vi "loop20 (Kopie).vi"() -> ()   [LabVIEW 2010]
uses:
  <vilib>/Utility/file.llb/Write To Spreadsheet File (DBL).vi
  <vilib>/Analysis/NI_AALBase.lvlib
panel:
  out "Phasen Error":dbl
  out "Phasen Mean":dbl
  out "Amplituden Error":dbl
  out "Amplituden Mean":dbl
  out "Phasen":dbl[](array[numeric])
  out "Amplituden":dbl[](array[numeric])
  out "data X":dbl format="%#_6e"
  out "data Y":dbl
  in  "mode (0)":i16
  in  "address string":string="19"
  out "Counter":dbl[](array[numeric])
  in  "Path":path
  out "error out":errorcluster
  in  "error in (no error)":errorcluster
  in  "Start":dbl format="%.2f"
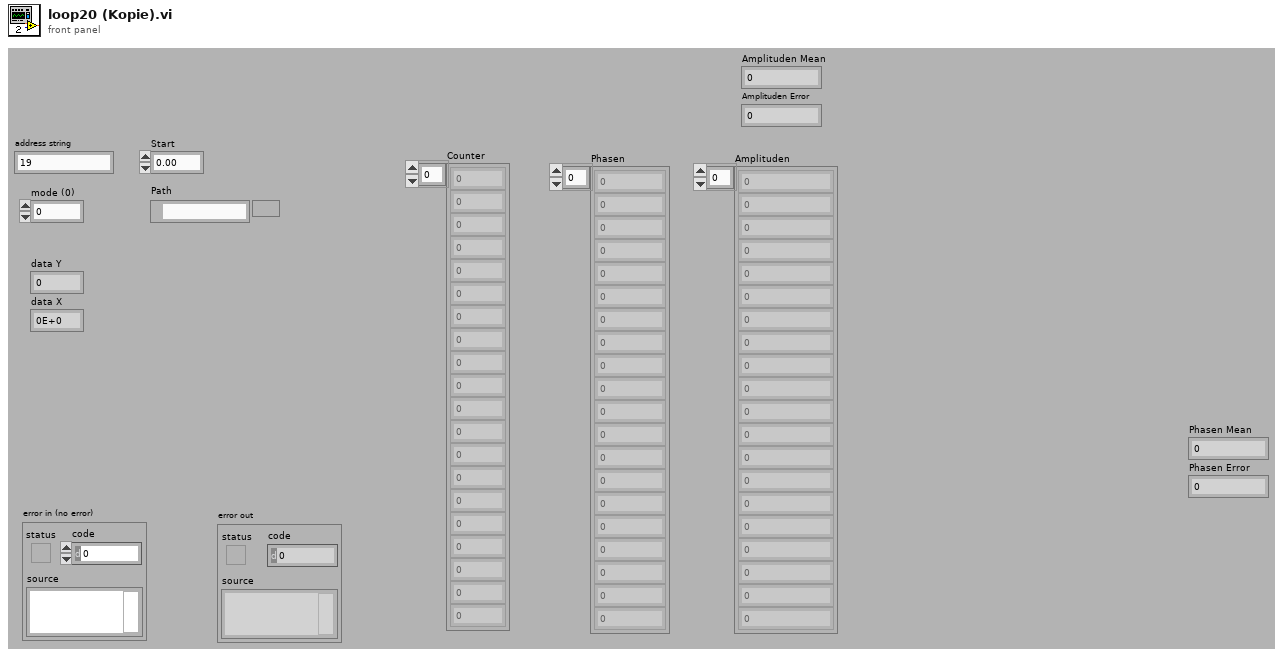
[diagram p1: front panel]
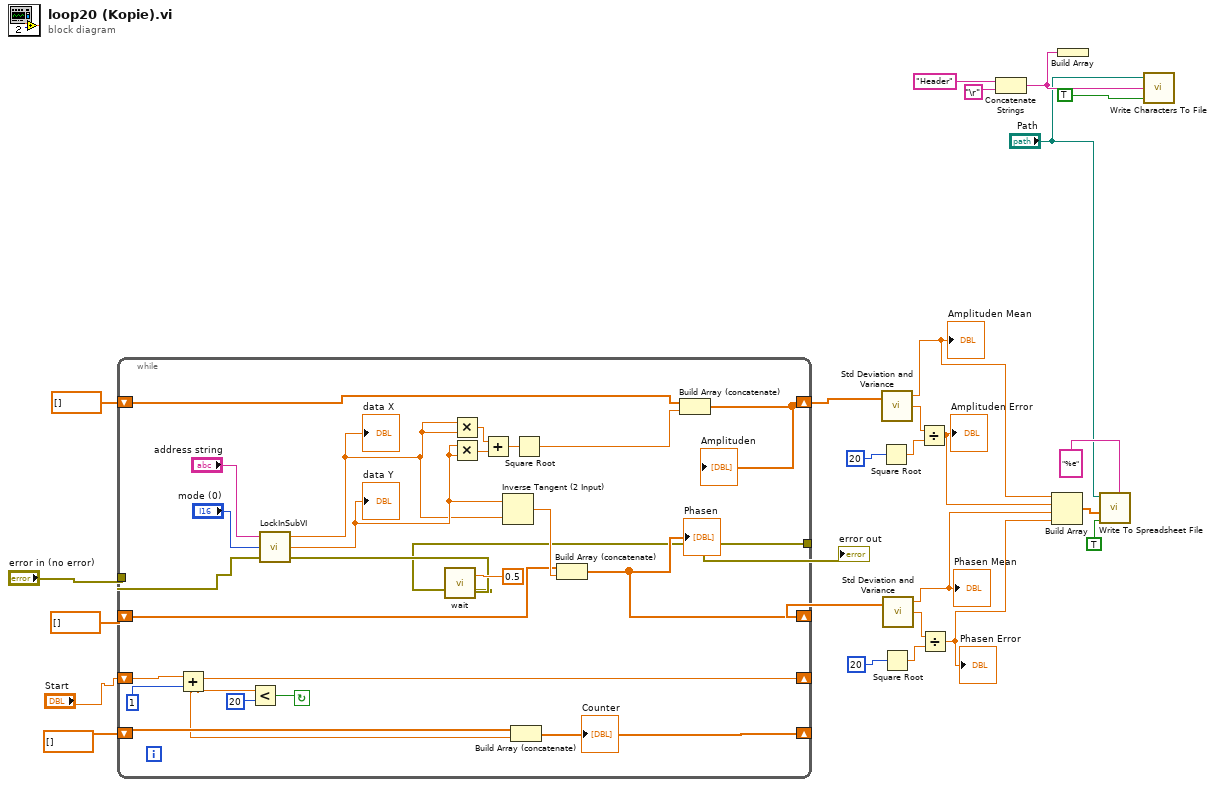
[diagram p0: block diagram]
diagram:
  n1 = while {
    tunnel: "error in (no error)" -> [w32]
    tunnel: [w33] -> w25
    shift-right: [w27] -> _
    shift-left: "Start" -> [w49]
    shift-right: [w28] -> _
    shift-left: dbl[] [] -> [w29]
    shift-right: [w39] -> w16
    shift-left: dbl[] [] -> [w40]
    shift-right: [w36] -> w9
    shift-left: dbl[] [] -> [w37]
    stop <- w30 continue-if-true
    n2 = Add(x=w49, y=1) -> (x+y=w27:dbl)
    n3 = Less?(x=w27, y=20) -> (x < y?=w30:bool)
    n4 = call "LockInSubVI.vi"("error in"=w32, "mode (0)"="mode (0)", "address string"="address string") -> ("error out 2"=w34:errorcluster, "data Y"=w43:dbl, "data X"=w42:dbl)
    "data Y" <- w43
    "data X" <- w42
    n5 = call "wait.vi"("error in"=w34, "Wartezeit in Sek"=0.5) -> ("error out"=w33:errorcluster)  [unwired: 1 in]
    n6 = Multiply(x=w42, y=w42) -> (x*y=w46:dbl)
    n7 = Multiply(x=w43, y=w43) -> (x*y=w45:dbl)
    n8 = Add(x=w46, y=w45) -> (x+y=w44:dbl)
    n9 = Inverse Tangent (2 Input)(1:w42, 2:w43) -> (0:w38:dbl)
    n10 = Build Array (concatenate)(w29, w27) -> (w28:dbl[])
    "Counter" <- w28
    n11 = Square Root(x=w44) -> (sqrt(x)=w41:dbl)
    n12 = Build Array (concatenate)(w37, w38) -> (w36:dbl[])
    "Phasen" <- w36
    n13 = Build Array (concatenate)(w40, w41) -> (w39:dbl[])
    "Amplituden" <- w39
  }
  "error out" <- w25
  n14 = Square Root(x=20) -> (sqrt(x)=w13:dbl)
  n15 = call <vilib>:"Std Deviation and Variance.vi"("X"=w16) -> ("mean"=w6:dbl, "standard deviation"=w15:dbl)  [unwired: 1 in, 1 out]
  "Amplituden Mean" <- w6
  n16 = Square Root(x=20) -> (sqrt(x)=w10:dbl)
  n17 = call <vilib>:"Std Deviation and Variance.vi"("X"=w9) -> ("mean"=w4:dbl, "standard deviation"=w12:dbl)  [unwired: 1 in, 1 out]
  "Phasen Mean" <- w4
  n18 = Divide(x=w15, y=w13) -> (x/y=w5:dbl)
  "Amplituden Error" <- w5
  n19 = Divide(x=w12, y=w10) -> (x/y=w3:dbl)
  "Phasen Error" <- w3
  n20 = Concatenate Strings("Header", "\r") -> (w21:string)
  n21 = Build Array(w6, w5, w4, w3) -> (w2:dbl[])
  n22 = Build Array(w21) -> ()  [unwired: 1 out]
  n23 = call-poly <vilib>:"Write To Spreadsheet File.vi"("format (%.3f)"="%e", "append to file? (new file:F)"=TRUE, "1D data"=w2, "file path (dialog if empty)"="Path") -> ()  [unwired: 4 in, 1 out]
  n24 = call <vilib>:"Write Characters To File.vi"("append to file? (new file:F)"=TRUE, "character string"=w21, "file path (dialog if empty)"="Path") -> ()  [unwired: 2 in, 1 out]
